vi "Pay.vi"(8 "error in (no error)":errorcluster, 10 "Accoounts":T1(c390), 11 "IAccountable in":refnum<class "IAccountable.lvclass">) -> (0 "error out":errorcluster, 2 "Accoounts out":T1(c390), 3 "IAccountable out":refnum<class "IAccountable.lvclass">)   [LabVIEW 2020, in "IAccountable.lvclass"]
uses:
  IAccountable.lvclass
  IBasicAccount/IBasicAccount.lvclass
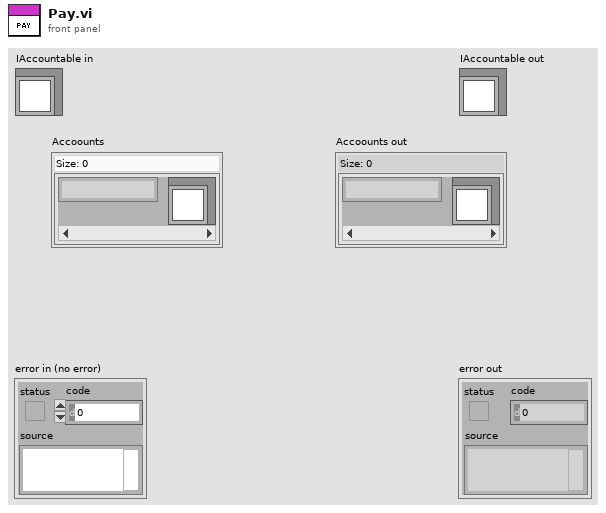
[diagram p1: front panel]
types:
  T1 = map{string, refnum<class "IBasicAccount.lvclass">}
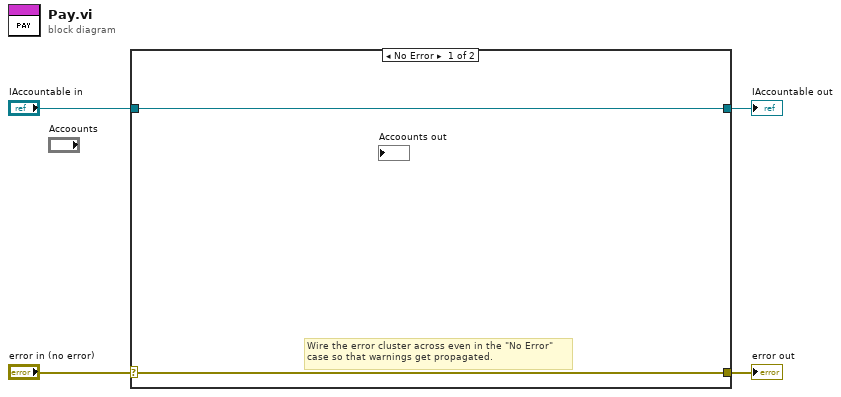
[diagram p0: block diagram]
diagram:
  n1 = case shown="No Error" "error in (no error)" {
    selector: "error in (no error)" -> [w5 w8]
    tunnel: [w5 w8] -> w3
    tunnel: [w6 w7] -> w1
    tunnel: "IAccountable in" -> [w6 w7]
    frame No Error {
      # "Wire the error cluster across even in the \"No Error\"\ncase so that warnings get propagated."
    }
    frame Error {
    }
  }
  "error out" <- w3
  "IAccountable out" <- w1
